vi "Get XY from player particle (SubVI).vi"(4 "Center of mass X":dbl, 5 "Image in Pixels (U8)":u8[][](array[numeric]), 6 "Particle bounding rect bottom":dbl, 7 "Particle bounding rect right":dbl, 8 "Particle bounding rect top":dbl, 9 "Particle bounding rect left":dbl) -> (0 "Y COM":i32, 1 "Y coordinate":i32, 2 "X coordinate":i32)   [LabVIEW 2014]
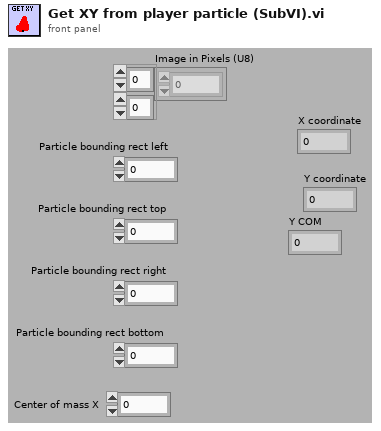
[diagram p1: front panel]
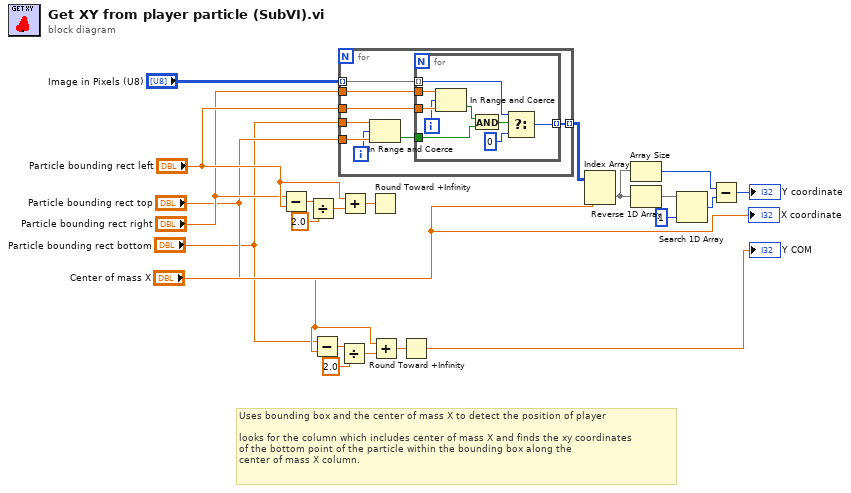
[diagram p0: block diagram]
diagram:
  # "Uses bounding box and the center of mass X to detect the position of player\n\nlooks for the column which includes center of mass X and finds the xy coordinates \nof the bottom point of the particle within the bounding box along the\ncenter of mass X column."
  n1 = Subtract(x="Particle bounding rect right", y="Particle bounding rect left") -> (x-y=w12:dbl)
  n2 = Divide(x=w12, y=2.0) -> (x/y=w15:dbl)
  n3 = Subtract(x="Particle bounding rect bottom", y="Particle bounding rect top") -> (x-y=w8:dbl)
  n4 = for {
    tunnel: "Image in Pixels (U8)" -> [w30] mode=indexing
    tunnel: "Particle bounding rect left" -> [w29]
    tunnel: "Particle bounding rect right" -> [w28]
    tunnel: "Particle bounding rect bottom" -> [w27]
    tunnel: "Particle bounding rect top" -> [w26]
    tunnel: [w23] -> w16 mode=indexing
    i -> [w25]
    n5 = In Range and Coerce(upper limit=w27, x=w25, lower limit=w26) -> (In Range?=w24:bool)  [unwired: 1 out]
    n6 = for {
      tunnel: w30 -> [w31] mode=indexing
      tunnel: w29 -> [w39]
      tunnel: w28 -> [w38]
      tunnel: w24 -> [w37]
      tunnel: [w33] -> w23 mode=indexing
      i -> [w32]
      n7 = In Range and Coerce(upper limit=w38, x=w32, lower limit=w39) -> (In Range?=w36:bool)  [unwired: 1 out]
      n8 = And(x=w36, y=w37) -> (x .and. y?=w35:bool)
      n9 = Select(t=w31, s=w35, f=u8 0) -> (s? t:f=w33:u8)
    }
  }
  n10 = Divide(x=w8, y=2.0) -> (x/y=w6:dbl)
  n11 = Add(x="Particle bounding rect left", y=w15) -> (x+y=w17:dbl)
  n12 = Round Toward +Infinity(x=w17) -> ()  [unwired: 1 out]
  n13 = Add(x="Particle bounding rect top", y=w6) -> (x+y=w5:dbl)
  n14 = Round Toward +Infinity(x=w5) -> (ceil(x): smallest int >= x=→"Y COM":dbl)
  n15 = Index Array(array=w16, index (col)="Center of mass X") -> (element=w18:u8[])  [unwired: 1 in]
  n16 = Array Size(array=w18) -> (size(s)=w21:i32)
  n17 = Reverse 1D Array(array=w18) -> (reversed array=w19:u8[])
  n18 = Search 1D Array(1D array=w19, element=u8 1) -> (index of element=w22:i32)  [unwired: 1 in]
  n19 = Subtract(x=w21, y=w22) -> (x-y=→"Y coordinate":i32)
  "X coordinate" <- "Center of mass X"
